vi "UIRefsSelector.vi"(10 "Enum 2":T1) -> (2 "String":string)   [LabVIEW 2014, in "UILib.lvlib"]
uses:
  UILib.lvlib
  UIRefs.ctl
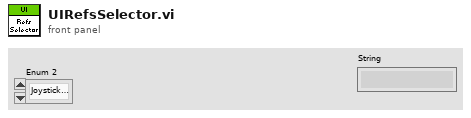
[diagram p1: front panel]
types:
  T1 = typedef "UILib.lvlib/UIRefs.ctl" = enum16{"Joystick0Ref"}
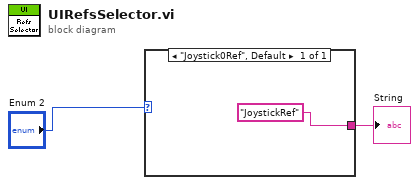
[diagram p0: block diagram]
diagram:
  n1 = case shown="\"Joystick0Ref\", Default" "Enum 2" {
    tunnel: ["JoystickRef"] -> w1
    frame "Joystick0Ref", Default {
    }
  }
  "String" <- w1
